vi "ImplementedDevices.vi"(11 "Index":i32) -> (0 "Not In List":bool, 1 "Menu Name":string, 3 "Device Out":refnum<class "Device.lvclass">)   [LabVIEW 2013]
doc: "Contains all implemented classes to appear in the Add Device menu, along with the text used to represent the device in said menu."
uses:
  Device/Device.lvclass
  DDS/DDS.lvclass
  Novatech/Novatech.lvclass
  NI Card/NI Card.lvclass
  Slave_Pulseblaster/Slave_Pulseblaster.lvclass
  PTS-via-PB/PTS-via-PB.lvclass
panel:
  # "To Add a device to the menu:\n- Go to the block diagram\n- Add a new case with the next numeric label\n- Connect the class to the \"Device Out\" terminal\n- Connect the menu entry to the \"Menu Name\" terminal\n- Connect a False boolean constant to the \"Not in List\" terminal"
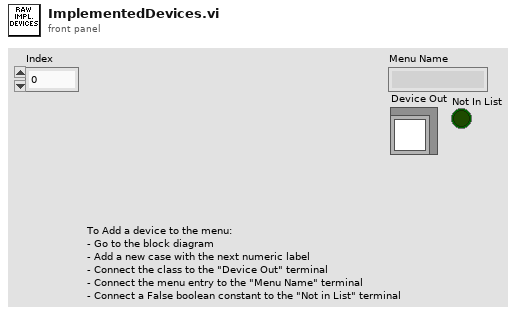
[diagram p1: front panel]
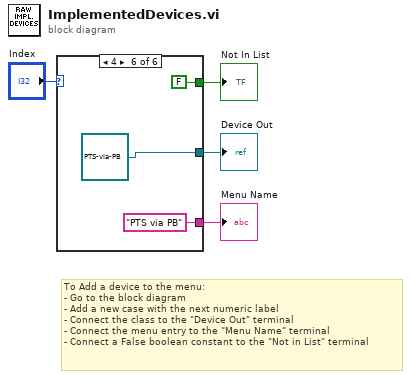
[diagram p0: block diagram]
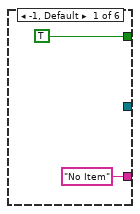
[diagram p2: hidden frame]
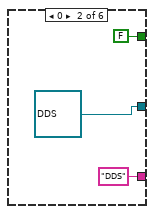
[diagram p3: hidden frame]
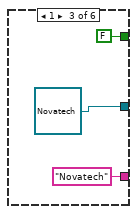
[diagram p4: hidden frame]
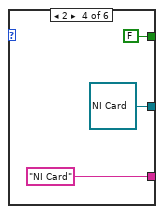
[diagram p5: hidden frame]
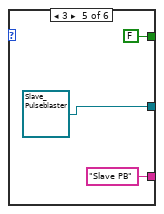
[diagram p6: hidden frame]
diagram:
  # "To Add a device to the menu:\n- Go to the block diagram\n- Add a new case with the next numeric label\n- Connect the class to the \"Device Out\" terminal\n- Connect the menu entry to the \"Menu Name\" terminal\n- Connect a False boolean constant to the \"Not in List\" terminal"
  n1 = case shown="4" "Index" {
    tunnel: ["No Item" "DDS" "Novatech" "NI Card" "Slave PB" "PTS via PB"] -> w3
    tunnel: [TRUE FALSE FALSE FALSE FALSE FALSE] -> w1
    tunnel: [_ refnum<class "DDS.lvclass"> refnum ("DDS.lvclass") refnum<class "Novatech.lvclass"> refnum ("Novatech.lvclass") refnum<class "NI Card.lvclass"> refnum ("NI Card.lvclass") refnum<class "Slave_Pulseblaster.lvclass"> refnum ("Slave_Pulseblaster.lvclass") refnum<class "PTS-via-PB.lvclass"> refnum ("PTS-via-PB.lvclass")] -> w2
    frame -1, Default {
    }
    frame 0 {
    }
    frame 1 {
    }
    frame 2 {
    }
    frame 3 {
    }
    frame 4 {
    }
  }
  "Menu Name" <- w3
  "Device Out" <- w2
  "Not In List" <- w1
